vi "MCL Grab Handle.vi"(11 "device":i16) -> (3 "function return":i32)   [LabVIEW 2017, in "Madlib.lvlib"]
doc: "MADLIB_API int MCL_GrabHandle(short device);"
uses:
  Madlib.lvlib
  Madlib.dll
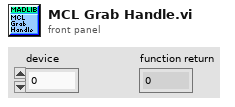
[diagram p1: front panel]
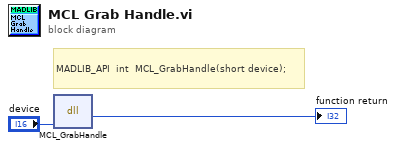
[diagram p0: block diagram]
diagram:
  # "MADLIB_API  int\t\tMCL_GrabHandle(short device);"
  n1 = dll-call lib="C:/Users/francesco/dev/pump-probe/Piezo/lvlib/Madlib.*" fn="MCL_GrabHandle"("device"="device") -> (→"function return":i32)  [unwired: 4 in, 2 out]
